vi "Update Current Index.vi"(5 "Display State In":T4={"Current Channels Info"=[], "Help Prefix"="", "Max Display Size"=8, "Max Size"=8, "Show Buttons"=TRUE, "Data Valid"=refnum, "Show Range"=FALSE, "Range Items"=[], "Range Index"=[]} caption="State", 7 "Channels In":T1, 8 "error in (no error)":errorcluster, 11 "Channels Reference":refnum<vi>) -> (0 "error out":errorcluster, 1 "Current Index":i32)   [LabVIEW 2021, in "myRIO Channel List.xctl"]
uses:
  <vilib>/myRIO/Common/Express VI Framework/xctls/myRIO Channel List/myRIO Channel List.xctl
  <vilib>/myRIO/Common/Express VI Framework/xctls/myRIO Channel List/State.ctl
  <vilib>/myRIO/Common/Profile Manager Framework/typedefs/Channel Info.ctl
  <vilib>/myRIO/Common/Express VI Framework/typedefs/Data Validate Ref.ctl
  <vilib>/myRIO/Common/Express VI Framework/xctls/myRIO Channel List/Data.ctl
  <vilib>/myRIO/Common/Express VI Framework/xctls/myRIO Channel List/typedefs/Channel Data.ctl
  <vilib>/myRIO/Common/Express VI Framework/xctls/myRIO Channel List/typedefs/Remove Channel.ctl
  <vilib>/myRIO/Common/Express VI Framework/xctls/myRIO Channel List/typedefs/Channel View.ctl
  <vilib>/myRIO/Common/Express VI Framework/xctls/myRIO Channel List/typedefs/Error Icon.ctl
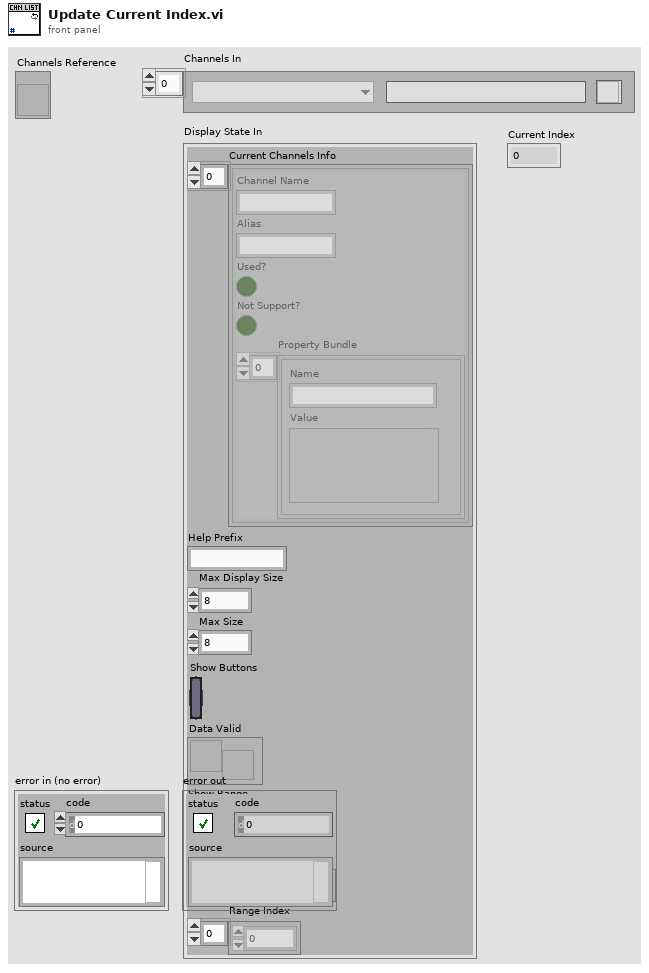
[diagram p1: front panel]
types:
  T1 = typedef "myRIO Channel List.xctl/Data.ctl" = T2[]
  T2 = typedef "myRIO Channel List.xctl/Channel Data.ctl" = cluster{"Channel Name":u16, "Channel Alias":string, "Remove Channel":T3, "Index":i32}
  T3 = typedef "myRIO Channel List.xctl/Remove Channel.ctl" = bool
  T4 = typedef "myRIO Channel List.xctl/State.ctl" = cluster{"Current Channels Info":T5[], "Help Prefix":string, "Max Display Size":i32, "Max Size":i32, "Show Buttons":bool, "Data Valid":T6, "Show Range":bool, "Range Items":string[], "Range Index":i32[]}
  T5 = typedef "Channel Info.ctl" = cluster{"Channel Name":string, "Alias":string, "Used?":bool, "Not Support?":bool, "Property Bundle":cluster{"Name":string, "Value":variant}[]}
  T6 = typedef "Data Validate Ref.ctl" = refnum<user-event>
  T7 = typedef "myRIO Channel List.xctl/Channel View.ctl" = cluster{"Error Icon":T8, "Channel Name":string, "Channel Alias":string, "Remove Channel":T3, "Index":i32, "Range":i32}
  T8 = typedef "myRIO Channel List.xctl/Error Icon.ctl" = bool
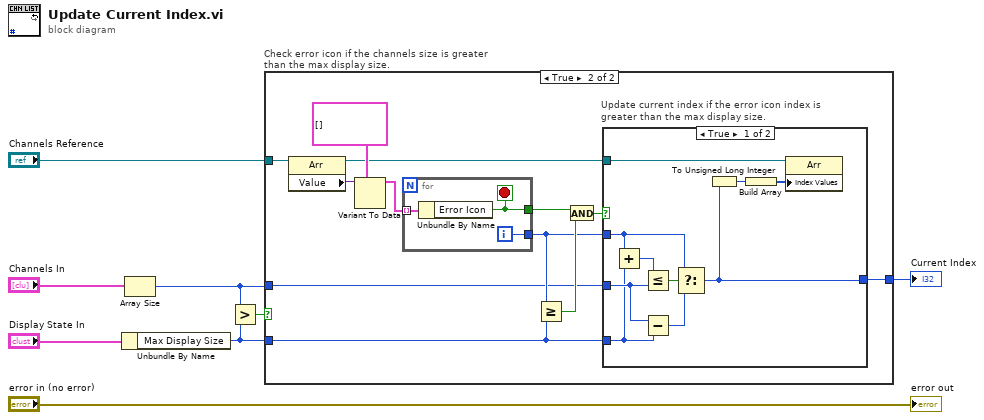
[diagram p0: block diagram]
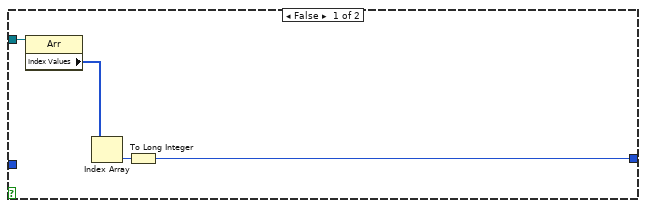
[diagram p2: hidden frame]
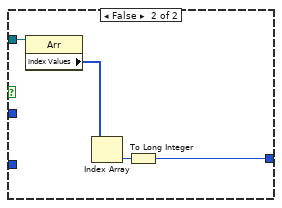
[diagram p3: hidden frame]
diagram:
  n1 = Unbundle By Name("Display State In") -> ("Max Display Size"=w6:i32)
  n2 = Array Size(array="Channels In") -> (size(s)=w7:i32)
  n3 = Greater?(x=w7, y=w6) -> (0:w8:bool)
  n4 = case "Check error icon if the channels size is greater than the max display size." shown="True" w8 {
    tunnel: "Channels Reference" -> [w12 w24]
    tunnel: w7 -> [_ w14]
    tunnel: w6 -> [_ w16]
    tunnel: [w9 w13] -> w5
    frame False {
      n5 = property class="Arr"(reference=w12) -> ("Index Values"=w11:u32[])  [unwired: 1 in, 2 out]
      n6 = Index Array(array=w11) -> (element=w10:u32)  [unwired: 1 in]
      n7 = To Long Integer(number=w10) -> (32bit integer=w9:i32)
    }
    frame True {
      n8 = property class="Arr"(reference=w24) -> (reference out=w20:refnum<vi>, "Value"=w23:variant)  [unwired: 1 in, 1 out]
      n9 = Variant To Data(type=T7[] [], Variant=w23) -> (data=w21:T7[])  [unwired: 1 in, 1 out]
      n10 = for {
        tunnel: w21 -> [w41] mode=indexing
        tunnel: [w40] -> w18
        tunnel: [w39] -> w15
        i -> [w39]
        stop <- w40 stop-if-true
        n11 = Unbundle By Name(w41) -> ("Error Icon"=w40:T8)
      }
      n12 = Greater Or Equal?(x=w15, y=w16) -> (x >= y?=w19:bool)
      n13 = And(x=w18, y=w19) -> (x .and. y?=w17:T8)
      n14 = case "Update current index if the error icon index is greater than the max display size." shown="True" w17 {
        tunnel: w20 -> [w28 w38]
        tunnel: w16 -> [w30 _]
        tunnel: w15 -> [w32 _]
        tunnel: w14 -> [w31 _]
        tunnel: [w27 w35] -> w13
        frame True {
          n15 = Add(x=w32, y=w30) -> (x+y=w34:i32)
          n16 = Less Or Equal?(x=w34, y=w31) -> (x <= y?=w33:bool)
          n17 = Subtract(x=w31, y=w30) -> (x-y=w29:i32)
          n18 = Select(t=w32, s=w33, f=w29) -> (s? t:f=w27:i32)
          n19 = To Unsigned Long Integer(number=w27) -> (unsigned 32bit integer=w25:u32)
          n20 = Build Array(w25) -> (w26:u32[])
          n21 = property class="Arr"(reference=w28, "Index Values"=w26) -> ()  [unwired: 1 in, 2 out]
        }
        frame False {
          n22 = property class="Arr"(reference=w38) -> ("Index Values"=w37:u32[])  [unwired: 1 in, 2 out]
          n23 = Index Array(array=w37) -> (element=w36:u32)  [unwired: 1 in]
          n24 = To Long Integer(number=w36) -> (32bit integer=w35:i32)
        }
      }
    }
  }
  "Current Index" <- w5
  "error out" <- "error in (no error)"
